vi "test - Get Status List.vi"(8 "error in (no error)":errorcluster, 11 "TestCase in":refnum<class "testcase-csmhelper.lvclass">) -> (0 "error out":errorcluster, 3 "TestCase out":refnum<class "testcase-csmhelper.lvclass">)   [LabVIEW 2017, in "testcase-csmhelper.lvclass"]
uses:
  testcase-csmhelper.lvclass
  src/user.lib/_NEVSTOP/Communicable State Machine(CSM)/_csmHelper/API/Create From VI Reference.vi
  src/user.lib/_NEVSTOP/Communicable State Machine(CSM)/_csmHelper/Properties/Read Status.vi
  <vilib>/addons/_JKI Toolkits/VI Tester/TestCase.llb/TestCase.lvclass
  src/user.lib/_NEVSTOP/Communicable State Machine(CSM)/_csmHelper/CSM-Helper.lvclass
  C:/Program Files (x86)/National Instruments/LabVIEW 2017/vi.lib/addons/_JKI Toolkits/VI Tester/TestCase.llb/TestCase.lvclass
panel:
  out "Array 3":cluster{"Status":string, "InState":string}[](array[cluster])
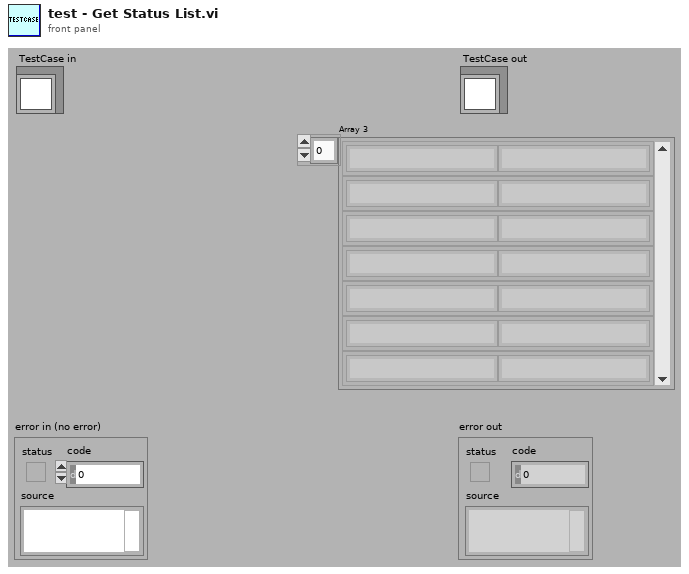
[diagram p1: front panel]
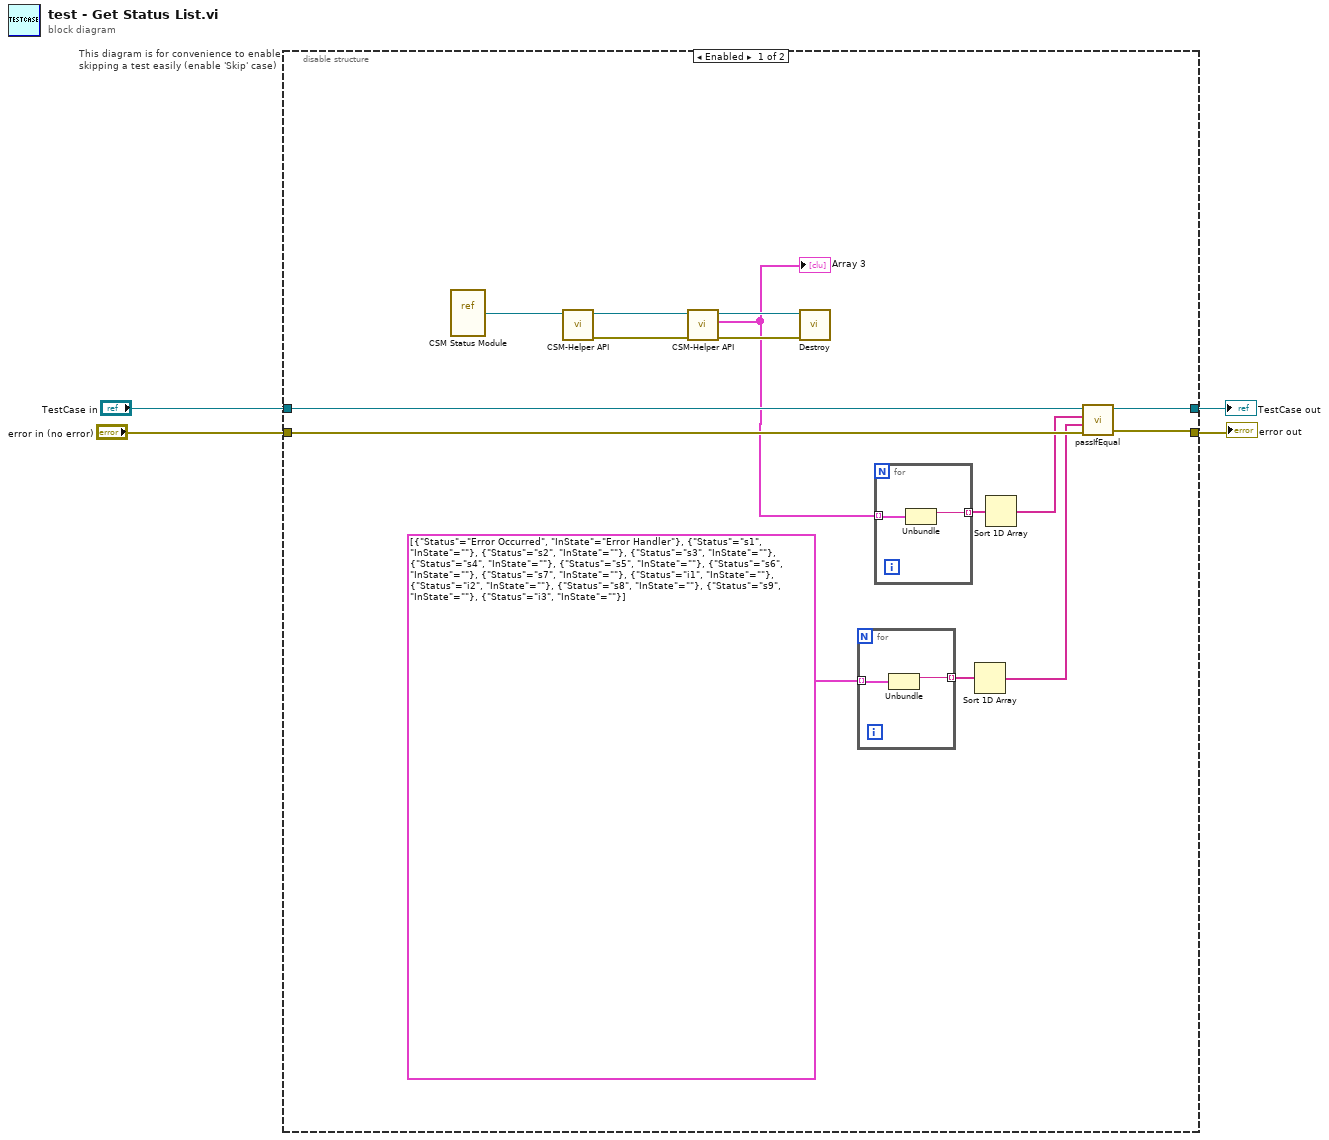
[diagram p0: block diagram]
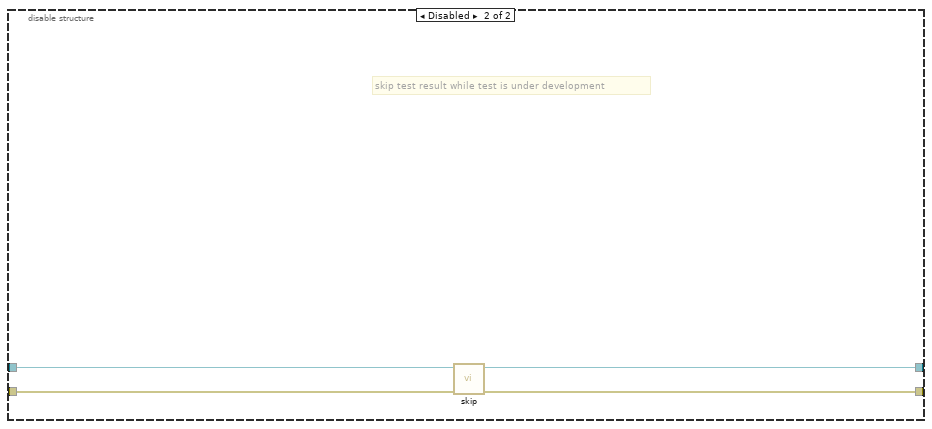
[diagram p2: hidden frame]
diagram:
  n1 = disable-structure "This diagram is for convenience to enable skipping a test easily (enable 'Skip' case)" shown="Enabled" {
    disable-tunnel: "TestCase in" -> [w19 w27]
    disable-tunnel: [w18 w25] -> w1
    disable-tunnel: [w17 w26] -> w3
    disable-tunnel: "error in (no error)" -> [w16 w24]
    frame Enabled {
      n2 = vi-ref "CSM Status Module.vi"() -> (w12:refnum<vi>)
      n3 = call-poly "CSM-Helper API.vi"("VI"=w12) -> ("error out"=w13:errorcluster, "CSM-Helper.lvclass"=w14:refnum<class "CSM-Helper.lvclass">)  [unwired: 9 in]
      n4 = call-poly "CSM-Helper API.vi"("error in (no error)"=w13, "CSM-Helper in"=w14) -> ("error out"=w11:errorcluster, "Array 3"=w9:cluster{"Status":string, "InState":string}[], "CSM-Helper out"=w15:refnum<class "CSM-Helper.lvclass">)  [unwired: 7 in]
      "Array 3" <- w9
      n5 = call "Destroy.vi"("error in (no error)"=w11, "CSM-Helper in"=w15) -> ()  [unwired: 8 in, 2 out]
      n6 = for {
        tunnel: cluster{"Status":string, "InState":string}[] [{"Status"="Error Occurred", "InState"="Error Handler"}, {"Status"="s1", "InState"=""}, {"Status"="s2", "InState"=""}, {"Status"="s3", "InState"=""}, {"Status"="s4", "InState"=""}, {"Status"="s5", "InState"=""}, {"Status"="s6", "InState"=""}, {"Status"="s7", "InState"=""}, {"Status"="i1", "InState"=""}, {"Status"="i2", "InState"=""}, {"Status"="s8", "InState"=""}, {"Status"="s9", "InState"=""}, {"Status"="i3", "InState"=""}] ("Array 3") -> [w23] mode=indexing
        tunnel: [w22] -> w7 mode=indexing
        n7 = Unbundle(w23) -> ("Status"=w22:string)  [unwired: 1 out]
      }
      n8 = for {
        tunnel: w9 -> [w21] mode=indexing
        tunnel: [w20] -> w8 mode=indexing
        n9 = Unbundle(w21) -> ("Status"=w20:string)  [unwired: 1 out]
      }
      n10 = Sort 1D Array(array=w7) -> (sorted array=w5:string[])
      n11 = Sort 1D Array(array=w8) -> (sorted array=w6:string[])
      n12 = call-dynamic "passIfEqual.vi"("error in (no error)"=w16, "y"=w5, "x"=w6, "TestCase in"=w19) -> ("error out"=w17:errorcluster, "TestCase out"=w18:refnum<class "testcase-csmhelper.lvclass">)  [unwired: 6 in]
    }
    frame Disabled {
      # "skip test result while test is under development"
      n13 = call <vilib>:"skip.vi"("error in (no error)"=w24, "TestCase in"=w27) -> ("error out"=w26:errorcluster, "TestCase out"=w25:refnum<class "testcase-csmhelper.lvclass">)  [unwired: 8 in]
    }
  }
  "error out" <- w3
  "TestCase out" <- w1
